vi "Send Message.vi"(4 "timeout in ms (100)":i32=100, 6 "ID":string, 8 "error in (no error)":errorcluster, 9 "Data":variant, 10 "Command":string, 11 "RemoteControl.ZMQ in":refnum<class "RemoteControl.ZMQ.lvclass">) -> (0 "error out":errorcluster, 2 "ACK":string, 3 "RemoteControl.ZMQ out":refnum<class "RemoteControl.ZMQ.lvclass">)   [LabVIEW 2019, in "RemoteControl.ZMQ.lvclass"]
uses:
  RemoteControl.ZMQ.lvclass
  C:/Users/patrick/Documents/GitHub/Instrument-Framework/lvsrc/SMOs/RemoteControl/RemoteControl.lvclass
  RemoteControl.ZMQ.lvclass/RemoteControl.ZMQ.ctl
  RemoteControl/Typedefs/Message--Cluster.ctl
  RemoteControl/RemoteControl.lvclass/RemoteControl.ctl
  <vilib>/addons/zeromq/zmq_socket.lvclass
  RemoteControl/RemoteControl.lvclass
  9a6b024f-cec4-4bd2-94ea-b4296ffc1878.vi
  3b72a26d-c3e2-4159-af9c-e2df9aaa681d.vi
  d8d7d812-ce68-4461-9032-ddc3f47440b3.vi
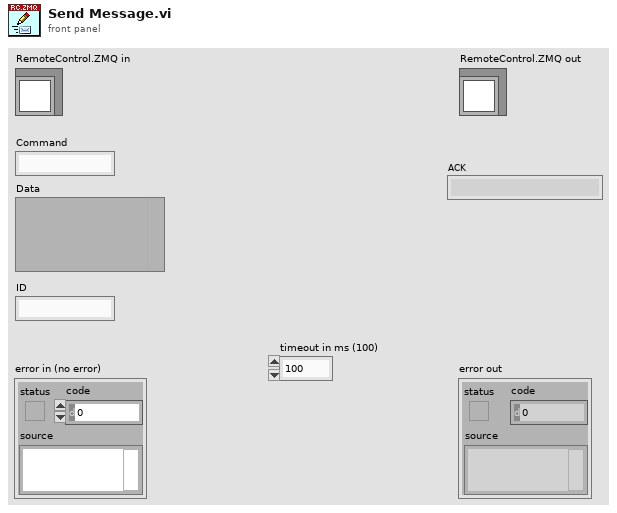
[diagram p1: front panel]
types:
  T1 = typedef "zeromq.lvlib/socket_type.ctl" = enum8{"ZMQ_PAIR", "ZMQ_PUB", "ZMQ_SUB", "ZMQ_REQ", "ZMQ_REP", "ZMQ_DEALER", "ZMQ_ROUTER", "ZMQ_PULL", "ZMQ_PUSH", "ZMQ_XPUB", "ZMQ_XSUB"}
  T2 = typedef "RemoteControl.lvclass/Message--Cluster.ctl" = cluster{"Command":string, "Data":variant, "ID":string}
  T3 = typedef "JSON-RPC.lvclass/Request--Cluster.ctl" = cluster{"method":string, "params":variant, "Notification?":bool}
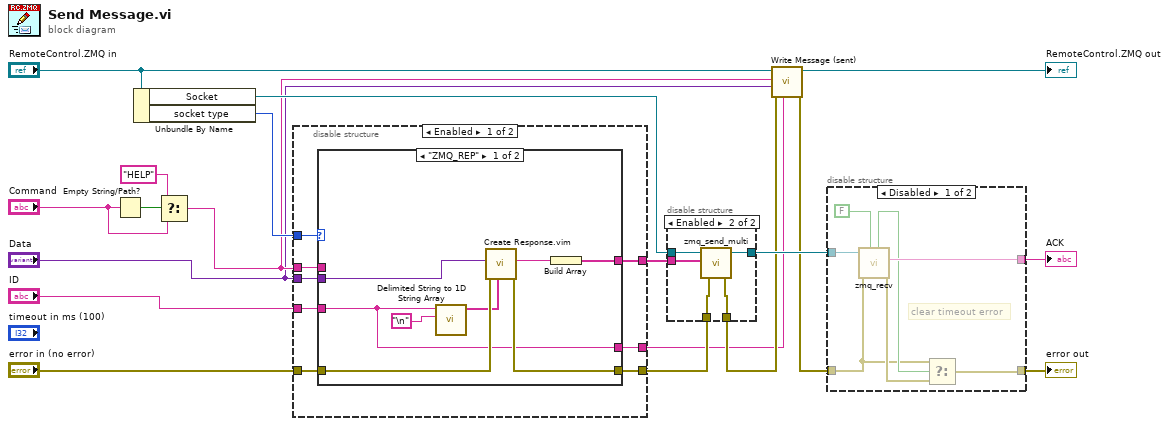
[diagram p0: block diagram]
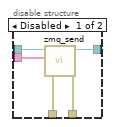
[diagram p2: hidden frame]
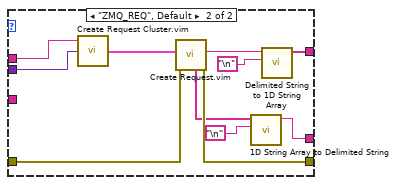
[diagram p3: hidden frame]
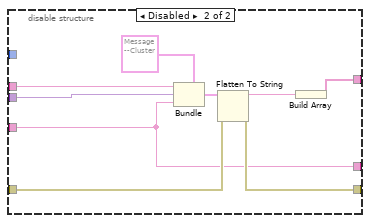
[diagram p4: hidden frame]
diagram:
  n1 = Empty String/Path?(string/path="Command") -> (empty?=w17:bool)
  n2 = Unbundle By Name("RemoteControl.ZMQ in") -> ("Socket"=w10:refnum<class "zmq_socket.lvclass">, "socket type"=w11:T1)
  n3 = Select(t="HELP", s=w17, f="Command") -> (s? t:f=w8:string)
  n4 = disable-structure shown="Enabled" {
    disable-tunnel: "Data" -> [w27 w49]
    disable-tunnel: w8 -> [w26 w50]
    disable-tunnel: [w25 w47] -> w7
    disable-tunnel: "error in (no error)" -> [w24 w53]
    disable-tunnel: [w23 w52] -> w13
    disable-tunnel: w11 -> [w22 _]
    disable-tunnel: "ID" -> [w20 w48]
    disable-tunnel: [w21 w48] -> w2
    frame Enabled {
      n5 = case shown="\"ZMQ_REP\"" w22 {
        tunnel: w26 -> [_ w40]
        tunnel: w27 -> [w35 w39]
        tunnel: [w28 w36] -> w25
        tunnel: w24 -> [w34 w45]
        tunnel: [w33 w44] -> w23
        tunnel: w20 -> [w30 _]
        tunnel: [w30 w41] -> w21
        frame "ZMQ_REP" {
          n6 = call <vilib>:"Delimited String to 1D String Array.vi"("delimiter"="\n", "delimited string"=w30) -> ("string array"=w31:string[])  [unwired: 9 in]
          n7 = call "Create Response.vim"("ids"=w31, "error in (no error)"=w34, "results"=w35) -> ("error out"=w33:errorcluster, "{JSON} Response"=w29:string)  [unwired: 6 in, 1 out]
          n8 = Build Array(w29) -> (w28:string[])
        }
        frame "ZMQ_REQ", Default {
          n9 = call "Create Request Cluster.vim"("params"=w39, "method"=w40) -> ("Requests"=w46:T3[])  [unwired: 1 in]
          n10 = call "Create Request.vim"("error in (no error)"=w45, "Requests"=w46) -> ("error out"=w44:errorcluster, "{JSON} Requests"=w37:string, "IDs"=w42:string[])  [unwired: 6 in, 1 out]
          n11 = call <vilib>:"1D String Array to Delimited String.vi"("delimiter"="\n", "string array"=w42) -> ("delimited string"=w41:string)  [unwired: 9 in]
          n12 = call <vilib>:"Delimited String to 1D String Array.vi"("delimiter"="\n", "delimited string"=w37) -> ("string array"=w36:string[])  [unwired: 9 in]
        }
      }
    }
    frame Disabled {
      n13 = Bundle(cluster=T2 {"Command"="", "Data"=variant, "ID"=""} ("Message"), "Command"=w50, "Data"=w49, "ID"=w48) -> (w55:T2)
      n14 = Flatten To String(anything=w55, error in (no error)=w53) -> (data string=w51:string, error out=w52:errorcluster)  [unwired: 2 in, 1 out]
      n15 = Build Array(w51) -> (w47:string[])
    }
  }
  n16 = disable-structure shown="Enabled" {
    disable-tunnel: [w60 w64] -> w16
    disable-tunnel: w13 -> [w59 w63]
    disable-tunnel: w10 -> [w58 w65]
    disable-tunnel: w7 -> [w57 w61]
    disable-tunnel: [w56 w62] -> w4
    frame Disabled {
      n17 = call <vilib>:"zmq_send.vi"("error in"=w59, "data"=w57, "socket in"=w58) -> ("error out"=w56:errorcluster, "socket out"=w60:refnum<class "zmq_socket.lvclass">)  [unwired: 4 in]
    }
    frame Enabled {
      n18 = call <vilib>:"zmq_send_multi.vi"("error in"=w63, "parts"=w61, "socket in"=w65) -> ("error out"=w62:errorcluster, "socket out"=w64:refnum<class "zmq_socket.lvclass">)  [unwired: 1 in]
    }
  }
  n19 = call "Write Message (sent).vi"("ID (sent)"=w2, "error in (no error)"=w4, "Data (sent)"="Data", "Command (sent)"=w8, "RemoteControl in"="RemoteControl.ZMQ in") -> ("error out"=w3:errorcluster, "RemoteControl out"=→"RemoteControl.ZMQ out":refnum<class "RemoteControl.ZMQ.lvclass">)  [unwired: 5 in]
  n20 = disable-structure shown="Disabled" {
    disable-tunnel: w16 -> [w72 _]
    disable-tunnel: [w71 _] -> w15
    disable-tunnel: [w67 w73] -> w12
    disable-tunnel: w3 -> [w66 w73]
    frame Disabled {
      # "clear timeout error"
      n21 = call <vilib>:"zmq_recv.vi"("no block? (F)"=FALSE, "error in"=w66, "socket in"=w72) -> ("error out"=w68:errorcluster, "data"=w71:string, "timeout?"=w69:bool)  [unwired: 2 in, 2 out]
      n22 = Select(t=w66, s=w69, f=w68) -> (s? t:f=w67:errorcluster)
    }
    frame Enabled {
    }
  }
  "error out" <- w12
  "ACK" <- w15
